vi "myRIO v1.0 AO Block Write.vi"(5 "Wait Until Done?":bool, 6 "AO FIFO Sample Rate":dbl=1000.0 min=1000.0 max=80000.0, 7 "Scale Constants Array":T1, 8 "error in (no error)":errorcluster, 9 "dbl Scaled Value List":dbl[][](array[numeric]), 10 "AO (N Samples) Channel List":T5, 11 "myRIO Ref In":T3) -> (0 "error out":errorcluster, 3 "myRIO Ref Out":T3)   [LabVIEW 2021]
uses:
  <vilib>/myRIO/Common/Instrument Driver Framework/myRIO v1.0/AO Block/typedefs/AO Block Channels List.ctl
  <vilib>/myRIO/Common/Instrument Driver Framework/myRIO v1.0/AO Block/typedefs/AO Block Channels Enum.ctl
  <vilib>/myRIO/Common/Instrument Driver Framework/Utilities/typedefs/myRIO v1.0 Reference.ctl
  <vilib>/myRIO/Common/Instrument Driver Framework/Utilities/typedefs/Generic FPGA Reference.ctl
  <vilib>/myRIO/Common/Instrument Driver Framework/Utilities/typedefs/Analog Scaling Constants List.ctl
  <vilib>/myRIO/Common/Instrument Driver Framework/Utilities/typedefs/Analog Scaling Constants.ctl
  <vilib>/myRIO/Common/Instrument Driver Framework/myRIO v1.0/AO Block/typedefs/AO Block Channels FPGA Reference.ctl
  <vilib>/myRIO/Common/Instrument Driver Framework/myRIO v1.0/AO Block/typedefs/AO Block Configuration.ctl
  <vilib>/myRIO/Common/Instrument Driver Framework/myRIO v1.0/Resource Manager/vis/myRIO v1.0 Block Write Configuration.vi
  <vilib>/rvi/errors/niLvFpgaAdjustHostInterfaceError.vi
  <vilib>/RVI Host/nirviSupport.llb/nirviErrorClusterFromErrorCode.vi
  <vilib>/rvi/interface/nirviReadWriteControl/nirviReadWriteControl.xnode
  <vilib>/rvi/interface/nirviMethod/nirviMethod.xnode
  <vilib>/rvi/interface/Simulation/niFpgaSimulationCallBeginRW.vi
  <vilib>/rvi/interface/nirviMethod/StockFPGA_InlinedMethodWaitForSingleIRQ.vi
  <vilib>/FPGAPlugInAG/Dynamic/niLvFpga_WaitOnIrq_Dynamic.vi
  <vilib>/FPGAPlugInAG/Dynamic/niLvFpga_AcknowledgeIrq_Dynamic.vi
  NiFpgaLv.dll
  <vilib>/FPGAPlugInAG/Dynamic/niLvFpga_WriteFifo_Dynamic.vi
  <vilib>/rvi/errors/niLvFpgaMergeErrorWithErrorCode.vi
panel:
  # "This VI writes  analog values to user specified analog output channels on the myRIO v1.0 hardware. The values are input as dbl values and scaled to u16 for input to the FPGA based on the specifications of the DAC. Please see Block Diagram for details."
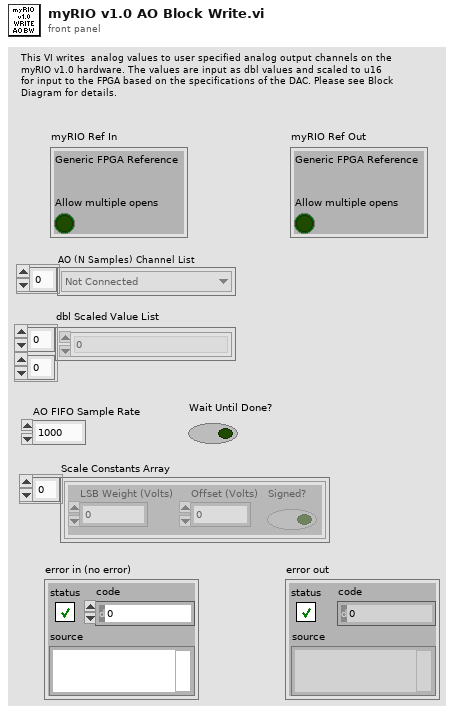
[diagram p1: front panel]
types:
  T1 = typedef "Analog Scaling Constants List.ctl" = T2[]
  T2 = typedef "Analog Scaling Constants.ctl" = cluster{"LSB Weight (Volts)":dbl, "Offset (Volts)":dbl, "Signed?":bool}
  T3 = typedef "myRIO v1.0 Reference.ctl" = cluster{"Generic FPGA Reference":T4, "Allow multiple opens":bool}
  T4 = typedef "Generic FPGA Reference.ctl" = refnum<k20>
  T5 = typedef "AO Block Channels List.ctl" = T6[]
  T6 = typedef "AO Block Channels Enum.ctl" = enum16{"Not Connected", "A/AO0 (N Samples)", "A/AO1 (N Samples)", "B/AO0 (N Samples)", "B/AO1 (N Samples)"}
  T7 = typedef "AO Block Channels FPGA Reference.ctl" = refnum<k20>
  T8 = typedef "AO Block Configuration.ctl" = cluster{"Wait Until Done?":bool, "AO FIFO Sample Rate(ticks)":u32, "Occurrence Handler ":refnum<k4>, "Analog data reference":refnum<data-value>}
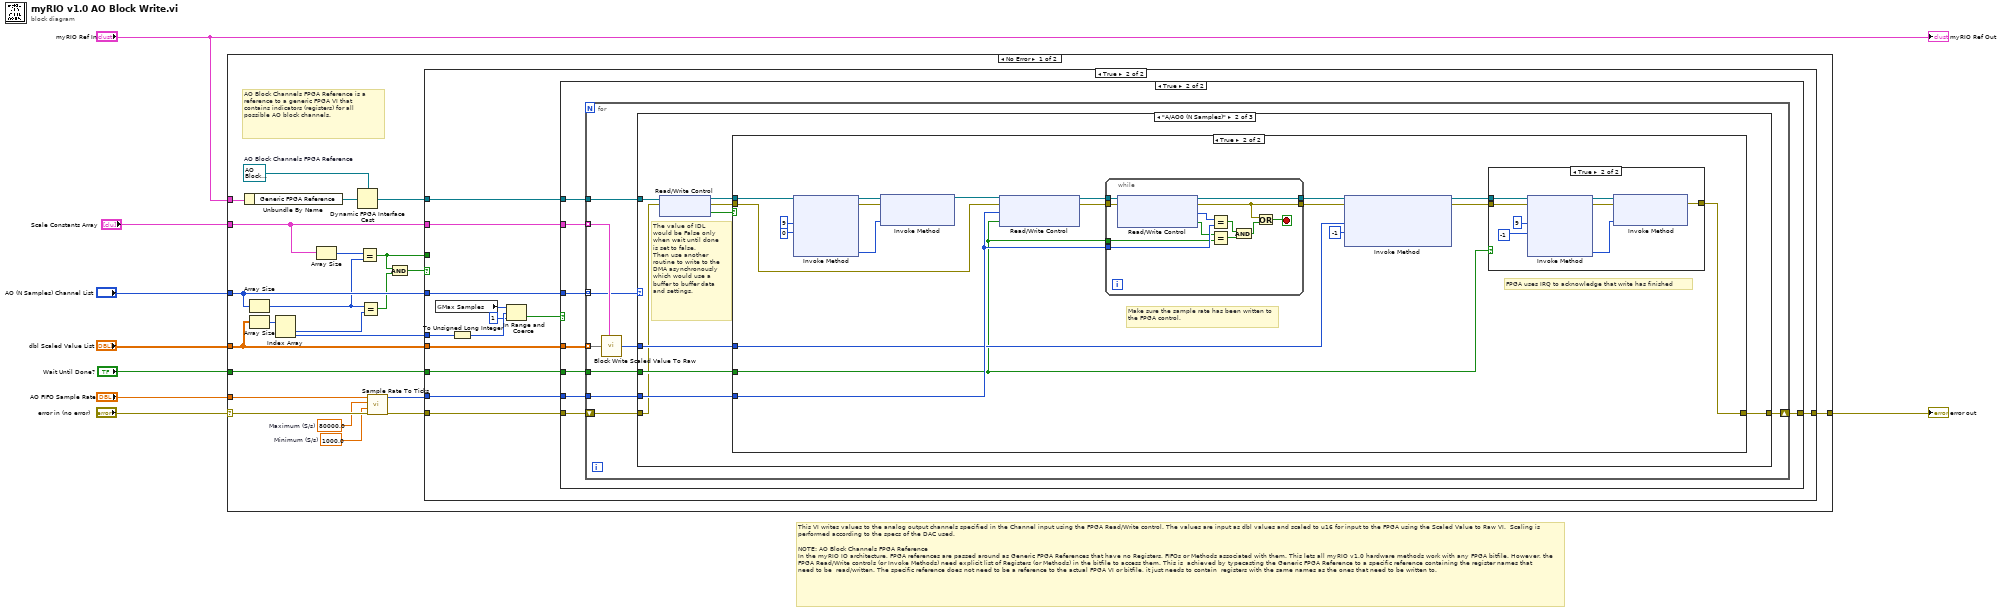
[diagram p0: block diagram]
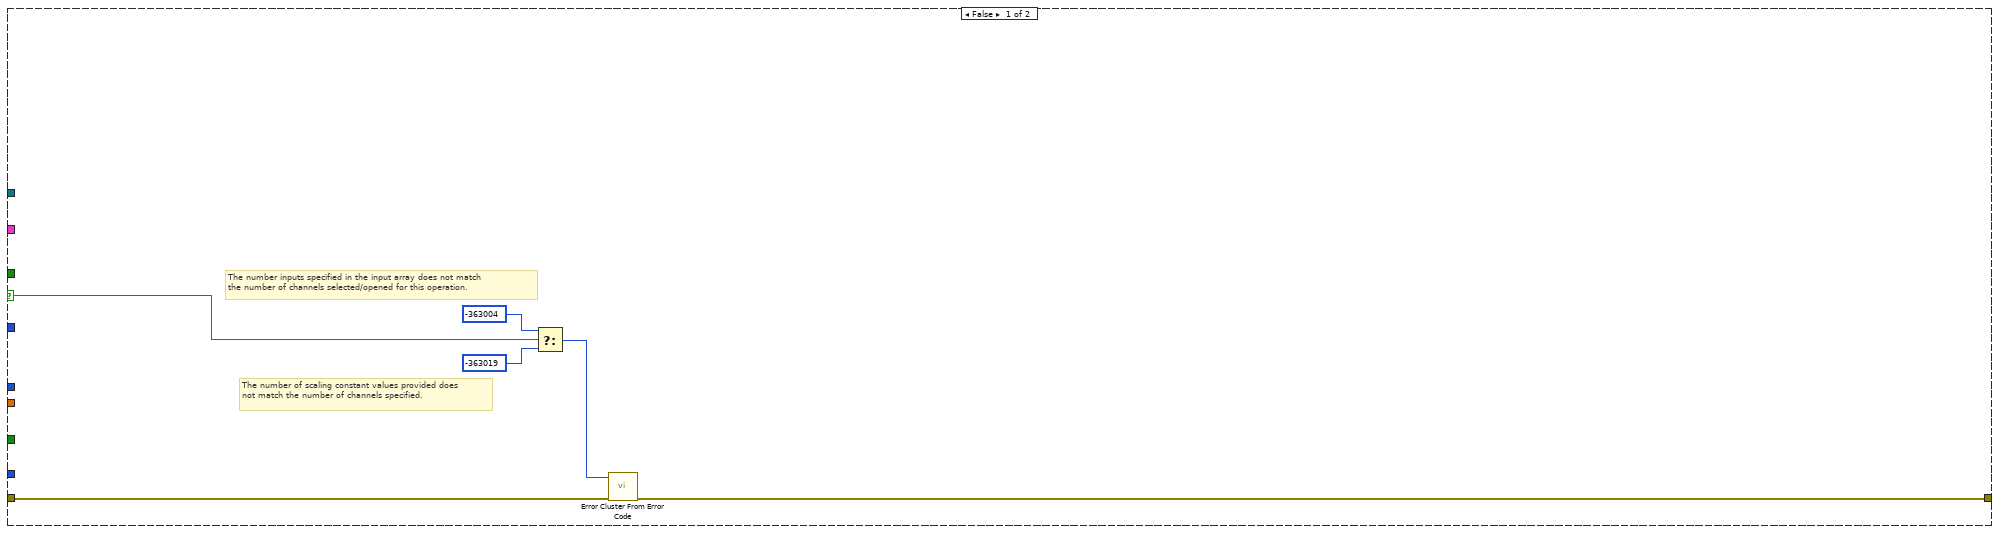
[diagram p2: hidden frame]
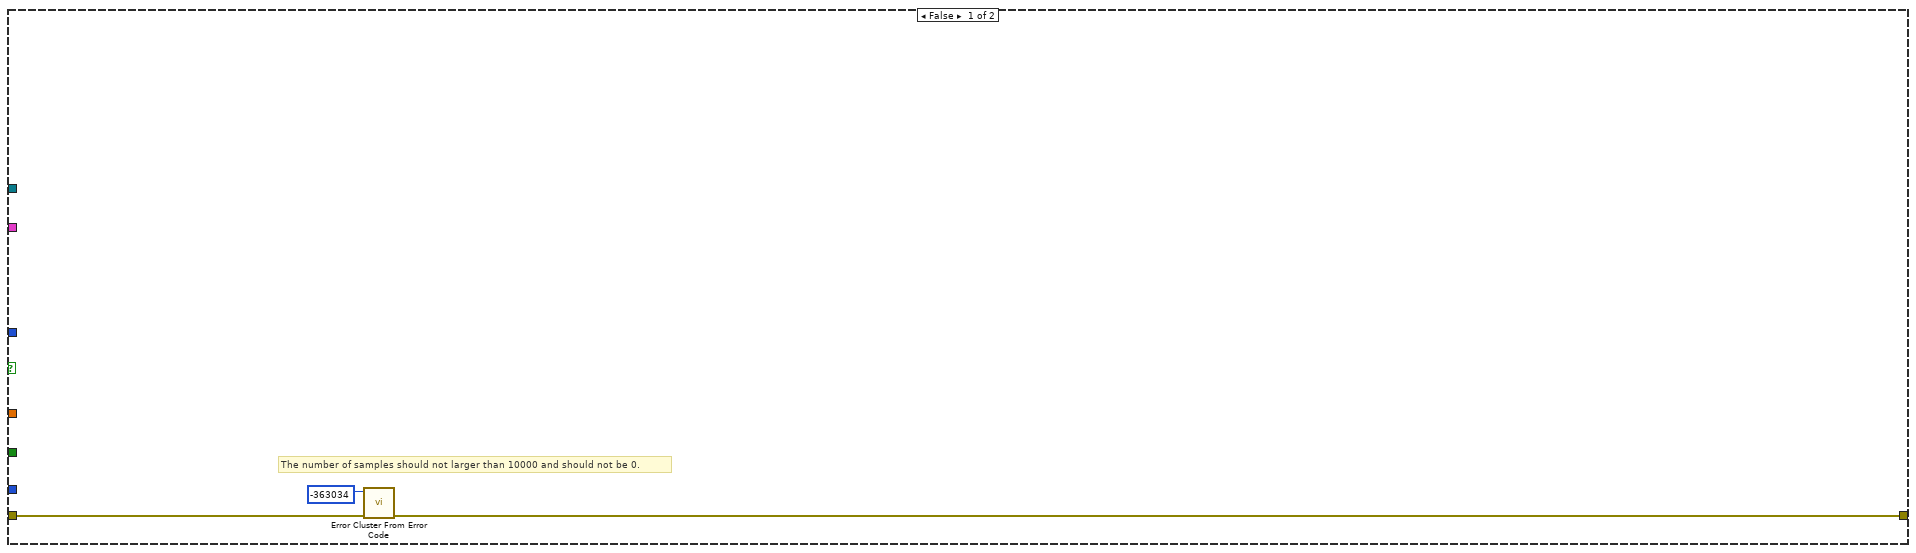
[diagram p3: hidden frame]
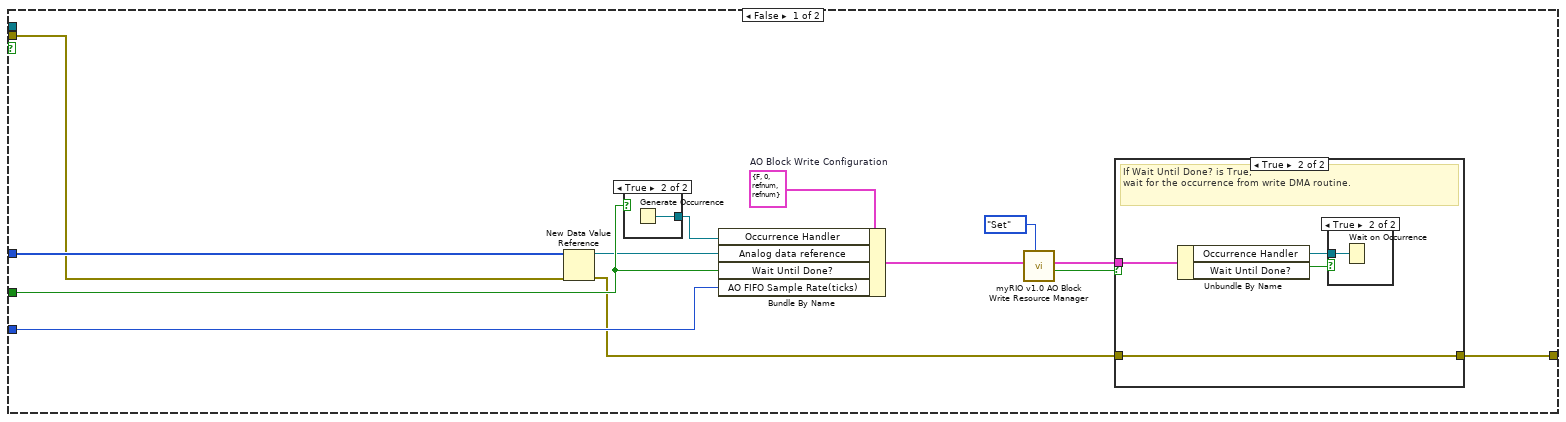
[diagram p5: hidden frame]
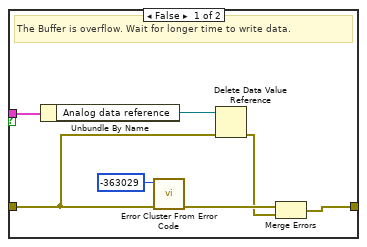
[diagram p6: hidden frame]
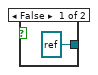
[diagram p8: hidden frame]
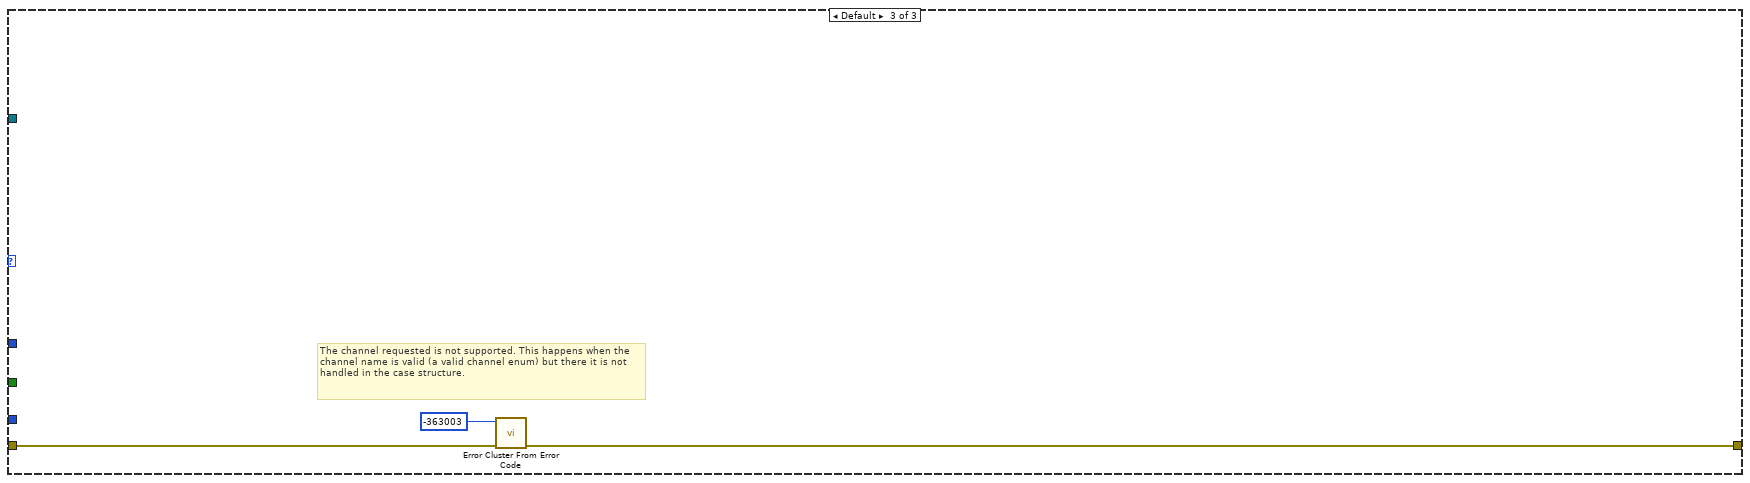
[diagram p10: hidden frame]
diagram:
  # "This VI writes values to the analog output channels specified in the Channel input using the FPGA Read/Write control. The values are input as dbl values and scaled to u16 for input to the FPGA using the Scaled Value to Raw VI.  Scaling is performed according to the specs of the DAC used.\n\nNOTE: AO Block Channels FPGA Reference\nIn the myRIO IO architecture, FPGA references are passed around as Generic FPGA References that have no Registers, FIFOs or Methods associated with them. This lets all myRIO v1.0 hardware methods work with any FPGA bitfile. However, the  FPGA Read/Write controls (or Invoke Methods) need explicit list of Registers (or Methods) in the bitfile to access them. This is  achieved by typecasting the Generic FPGA Reference to a specific reference containing the register names that need to be  read/written. The specific reference does not need to be a reference to the actual FPGA VI or bitfile, it just needs to contain  registers with the same names as the ones that need to be written to."
  n1 = case shown="No Error" "error in (no error)" {
    selector: "error in (no error)" -> [w11 w151]
    tunnel: [w31 w151] -> w8
    tunnel: "AO (N Samples) Channel List" -> [w30 _]
    tunnel: "dbl Scaled Value List" -> [w29 _]
    tunnel: "AO FIFO Sample Rate" -> [w14 _]
    tunnel: "Scale Constants Array" -> [w24 _]
    tunnel: "Wait Until Done?" -> [w23 _]
    tunnel: "myRIO Ref In" -> [w20 _]
    frame No Error {
      w9 = 1000.0  # Minimum (S/s)
      w10 = 80000.0  # Maximum (S/s)
      w18 = T7 refnum  # AO Block Channels FPGA Reference
      # "AO Block Channels FPGA Reference is a reference to a generic FPGA VI that contains indicators (registers) for all possible AO block channels."
      n2 = Unbundle By Name(w20) -> ("Generic FPGA Reference"=w21:T4)
      n3 = Array Size(array=w30) -> (size(s)=w26:i32)
      n4 = Array Size(array=w29) -> (size(s)=w28:i32[])
      n5 = Index Array(array=w28) -> (element #1=w16:i32, element #2=w15:i32)  [unwired: 2 in]
      n6 = Array Size(array=w24) -> (size(s)=w27:i32)
      n7 = Dynamic FPGA Interface Cast(Session In=w18, Type=w21) -> (Session Out=w19:T7)
      n8 = Equal?(x=w27, y=w26) -> (x = y?=w17:bool)
      n9 = Equal?(x=w26, y=w16) -> (x = y?=w25:bool)
      n10 = call <vilib>:"Sample Rate To Ticks.vi"("error in (no error)"=w11, "Minimum (S/s)"=w9, "Maximum (S/s)"=w10, "Sample Rate (S/s)"=w14) -> ("error out"=w12:errorcluster, "Count (tick/s)"=w13:u32)  [unwired: 5 in, 1 out]
      n11 = And(x=w17, y=w25) -> (x .and. y?=w22:bool)
      n12 = case shown="True" w22 {
        selector: w22 -> [w32 _]
        tunnel: [w37 w47] -> w31
        tunnel: w30 -> [_ w49]
        tunnel: w29 -> [_ w48]
        tunnel: w17 -> [_ _]
        tunnel: w24 -> [_ w50]
        tunnel: w23 -> [_ w46]
        tunnel: w19 -> [_ w45]
        tunnel: w15 -> [_ w44]
        tunnel: w13 -> [_ w43]
        tunnel: w12 -> [w33 w42]
        frame False {
          # "The number of scaling constant values provided does not match the number of channels specified."
          # "The number inputs specified in the input array does not match\nthe number of channels selected/opened for this operation."
          n13 = Select(t=-363004 ("error code (0)"), s=w32, f=-363019 ("error code (0)")) -> (s? t:f=w34:i32)
          n14 = call <vilib>:"Error Cluster From Error Code.vi"("error in (no error)"=w33, "error code (0)"=w34) -> ("error out"=w37:errorcluster)  [unwired: 7 in]
        }
        frame True {
          n15 = global read "myRIO v1.0 Block Write Configuration.vi" "Max Samples"() -> (w41:u32)
          n16 = To Unsigned Long Integer(number=w44) -> (unsigned 32bit integer=w40:u32)
          n17 = In Range and Coerce(upper limit=w41, x=w40, lower limit=u32 1) -> (In Range?=w38:bool)  [unwired: 1 out]
          n18 = case shown="True" w38 {
            tunnel: w50 -> [_ w61]
            tunnel: w49 -> [_ w60]
            tunnel: w48 -> [_ w59]
            tunnel: [w53 w58] -> w47
            tunnel: w46 -> [_ w57]
            tunnel: w45 -> [_ w56]
            tunnel: w43 -> [_ w55]
            tunnel: w42 -> [w51 w54]
            frame False {
              # "The number of samples should not larger than 10000 and should not be 0."
              n19 = call <vilib>:"Error Cluster From Error Code.vi"("error in (no error)"=w51, "error code (0)"=-363034) -> ("error out"=w53:errorcluster)  [unwired: 7 in]
            }
            frame True {
              n20 = for {
                tunnel: w59 -> [w69] mode=indexing
                tunnel: w60 -> [w65] mode=indexing
                shift-right: [w70] -> w58
                shift-left: w54 -> [w62]
                tunnel: w61 -> [w67] mode=indexing
                tunnel: w57 -> [w66]
                tunnel: w56 -> [w64]
                tunnel: w55 -> [w63]
                n21 = call <vilib>:"Block Write Scaled Value To Raw.vi"("Scaling Constants"=w67, "dbl Scaled Value"=w69) -> ("u16 Raw Value"=w68:u16[])  [unwired: 7 in]
                n22 = case shown="\"A/AO0 (N Samples)\"" w65 {
                  tunnel: w62 -> [w71 w73 w149]
                  tunnel: [w71 w77 w148] -> w70
                  tunnel: w68 -> [_ w80 _]
                  tunnel: w63 -> [_ w78 _]
                  tunnel: w66 -> [_ w79 _]
                  tunnel: w64 -> [_ w76 _]
                  frame "Not Connected" {
                  }
                  frame "A/AO0 (N Samples)" {
                    # "The value of IDL\nwould be False only \nwhen wait until done\nis set to false.\nThen use another \nroutine to write to the \nDMA asynchronously\nwhich would use a \nbuffer to buffer data \nand settings."
                    n23 = xnode "Read/Write Control"("FPGA VI Reference In"=w76, "error in"=w73) -> ("FPGA VI Reference Out"=w75:T7, "error out"=w74:errorcluster, "AO.A_0.IDL"=w72:bool)
                    n24 = case shown="True" w72 {
                      tunnel: w80 -> [w93 w109]
                      tunnel: w79 -> [w92 w108]
                      tunnel: w78 -> [w91 w124]
                      tunnel: [w90 w118] -> w77
                      tunnel: w74 -> [w88 w110]
                      tunnel: w75 -> [_ w111]
                      frame False {
                        w85 = T8 {"Wait Until Done?"=FALSE, "AO FIFO Sample Rate(ticks)"=0, "Occurrence Handler "=refnum, "Analog data reference"=refnum}  # AO Block Write Configuration
                        n25 = New Data Value Reference(data value=w93, error in=w88) -> (data value reference=w87:refnum<data-value>, error out=w89:errorcluster)
                        n26 = case shown="True" w92 {
                          tunnel: [refnum<k4> refnum ("occurrence") w107] -> w86
                          frame False {
                          }
                          frame True {
                            n27 = Generate Occurrence() -> (w107:refnum<k4>)
                          }
                        }
                        n28 = Bundle By Name(cluster=w85, "Occurrence Handler"=w86, "Analog data reference"=w87, "Wait Until Done?"=w92, "AO FIFO Sample Rate(ticks)"=w91) -> (w82:T8)
                        n29 = call <vilib>:"myRIO v1.0 AO Block Write Resource Manager.vi"("Action"=enum16{"Get", "Set"}."Set", "AO Resource In"=w82) -> ("Action Succeeds"=w84:bool, "AO Resource Out"=w81:T8)  [unwired: 8 in]
                        n30 = case shown="True" w84 {
                          tunnel: w89 -> [w97 w104]
                          tunnel: [w94 w104] -> w90
                          tunnel: w81 -> [w99 w101]
                          frame False {
                            # "The Buffer is overflow. Wait for longer time to write data."
                            n31 = Unbundle By Name(w99) -> ("Analog data reference"=w98:refnum<data-value>)
                            n32 = call <vilib>:"Error Cluster From Error Code.vi"("error in (no error)"=w97, "error code (0)"=-363029) -> ("error out"=w96:errorcluster)  [unwired: 7 in]
                            n33 = Delete Data Value Reference(data value reference=w98, error in=w97) -> (error out=w95:errorcluster)  [unwired: 1 out]
                            n34 = Merge Errors(w96, w95) -> (w94:errorcluster)
                          }
                          frame True {
                            # "If Wait Until Done? is True, \nwait for the occurrence from write DMA routine."
                            n35 = Unbundle By Name(w101) -> ("Occurrence Handler"=w102:refnum<k4>, "Wait Until Done?"=w103:bool)
                            n36 = case shown="True" w103 {
                              tunnel: w102 -> [_ w105]
                              frame False {
                              }
                              frame True {
                                n37 = Wait on Occurrence(2:w105) -> ()  [unwired: 2 in, 1 out]
                              }
                            }
                          }
                        }
                      }
                      frame True {
                        # "Make sure the sample rate has been written to the FPGA control."
                        # "FPGA uses IRQ to acknowledge that write has finished"
                        n38 = xnode "Invoke Method"("FPGA VI Reference In"=w111, "IRQ Number(s)"=9, "Timeout (ms)"=0) -> ("FPGA VI Reference Out"=w115:T7, "error out"=w116:errorcluster, "IRQ(s) Asserted"=w117:i32)  [unwired: 1 in, 1 out]
                        n39 = xnode "Invoke Method"("FPGA VI Reference In"=w115, "error in"=w116, "IRQ Number(s)"=w117) -> ("FPGA VI Reference Out"=w112:T7)  [unwired: 1 out]
                        n40 = xnode "Read/Write Control"("FPGA VI Reference In"=w112, "error in"=w110, "AO.A_0.SampleRate"=w124, "AO.A_0.IRQ.SELECT"=w108) -> ("FPGA VI Reference Out"=w126:T7, "error out"=w125:errorcluster)
                        n41 = while {
                          tunnel: w126 -> [w147]
                          tunnel: [w146] -> w123
                          tunnel: [w142] -> w122
                          tunnel: w125 -> [w145]
                          tunnel: w124 -> [w144]
                          tunnel: w108 -> [w139]
                          stop <- w141 stop-if-true
                          n42 = xnode "Read/Write Control"("FPGA VI Reference In"=w147, "error in"=w145) -> ("FPGA VI Reference Out"=w146:T7, "error out"=w142:errorcluster, "AO.A_0.SampleRate"=w143:u32, "AO.A_0.IRQ.SELECT"=w140:bool)
                          n43 = Equal?(x=w143, y=w144) -> (x = y?=w137:bool)
                          n44 = Equal?(x=w140, y=w139) -> (x = y?=w138:bool)
                          n45 = And(x=w137, y=w138) -> (x .and. y?=w136:bool)
                          n46 = Or(x=w142, y=w136) -> (x .or. y?=w141:bool)
                        }
                        n47 = xnode "Invoke Method"("FPGA VI Reference In"=w123, "error in"=w122, "Data"=w109, "Timeout (ms)"=-1) -> ("FPGA VI Reference Out"=w120:T7, "error out"=w119:errorcluster)  [unwired: 1 out]
                        n48 = case shown="True" w108 {
                          tunnel: w120 -> [_ w134]
                          tunnel: w119 -> [w127 w133]
                          tunnel: [w127 w129] -> w118
                          frame False {
                          }
                          frame True {
                            n49 = xnode "Invoke Method"("FPGA VI Reference In"=w134, "error in"=w133, "IRQ Number(s)"=9, "Timeout (ms)"=-1) -> ("FPGA VI Reference Out"=w132:T7, "error out"=w131:errorcluster, "IRQ(s) Asserted"=w130:i32)  [unwired: 1 out]
                            n50 = xnode "Invoke Method"("FPGA VI Reference In"=w132, "error in"=w131, "IRQ Number(s)"=w130) -> ("error out"=w129:errorcluster)  [unwired: 1 out]
                          }
                        }
                      }
                    }
                  }
                  frame Default {
                    # "The channel requested is not supported. This happens when the channel name is valid (a valid channel enum) but there it is not handled in the case structure."
                    n51 = call <vilib>:"Error Cluster From Error Code.vi"("error in (no error)"=w149, "error code (0)"=-363003) -> ("error out"=w148:errorcluster)  [unwired: 7 in]
                  }
                }
              }
            }
          }
        }
      }
    }
    frame Error {
      # "There is an incoming error so there is nothing to do."
    }
  }
  "error out" <- w8
  "myRIO Ref Out" <- "myRIO Ref In"
